vi "Get All Addresses in a Generation.vi"(8 "error in":errorcluster, 10 "Generation":i32, 11 "XML Document in":refnum<class "XML Document.lvclass">) -> (0 "error out":errorcluster, 2 "Addresses":i32[][](array[numeric]), 3 "XML Document out":refnum<class "XML Document.lvclass">)   [LabVIEW 2014, in "XML Document.lvclass"]
uses:
  XML Document.lvclass
  Node_class/Node.lvclass
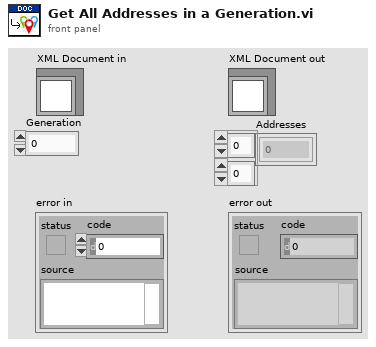
[diagram p1: front panel]
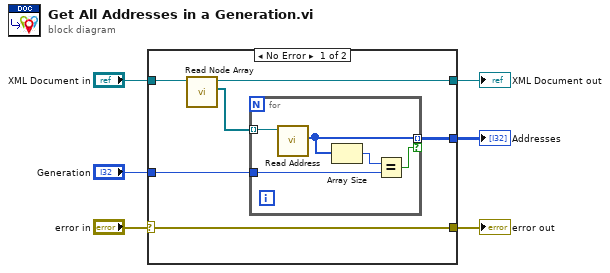
[diagram p0: block diagram]
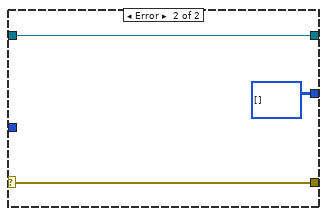
[diagram p2: hidden frame]
diagram:
  n1 = case shown="No Error" "error in" {
    selector: "error in" -> [w11 w20]
    tunnel: [w11 w20] -> w5
    tunnel: [w10 w19] -> w3
    tunnel: "XML Document in" -> [w12 w19]
    tunnel: "Generation" -> [w8 _]
    tunnel: [w7 i32[][] [] ("Address")] -> w1
    frame No Error {
      n2 = call-dynamic "Read Node Array.vi"("XML Document in"=w12) -> ("Node Array"=w9:refnum<class "Node.lvclass">[], "XML Document out"=w10:refnum<class "XML Document.lvclass">)  [unwired: 8 in, 1 out]
      n3 = for {
        tunnel: w9 -> [w17] mode=indexing
        tunnel: w8 -> [w15]
        tunnel: [w14] -> w7 mode=indexing if=w13
        n4 = call-dynamic "Read Address.vi"("Node in"=w17) -> ("Address"=w14:i32[])  [unwired: 8 in, 2 out]
        n5 = Array Size(array=w14) -> (size(s)=w16:i32)
        n6 = Equal?(x=w16, y=w15) -> (x = y?=w13:bool)
      }
    }
    frame Error {
    }
  }
  "error out" <- w5
  "XML Document out" <- w3
  "Addresses" <- w1
